vi "Set_PackedLibrary_Data.vi"(8 "error in (no error)":errorcluster, 10 "data":T1, 11 "Class in":refnum<class "AB_PackedLibrary.lvclass">) -> (0 "error out":errorcluster, 3 "Class out":refnum<class "AB_PackedLibrary.lvclass">)   [LabVIEW 2020, in "AB_PackedLibrary.lvclass"]
uses:
  <vilib>/AppBuilder/AB_Classes/PackedLib/AB_PackedLibrary.lvclass
  <vilib>/AppBuilder/AB_Classes/PackedLib/AB_PackedLibrary.ctl
  <vilib>/AppBuilder/AB_Classes/PackedLib/AB_PackedLibrary.lvclass/AB_PackedLibrary.ctl
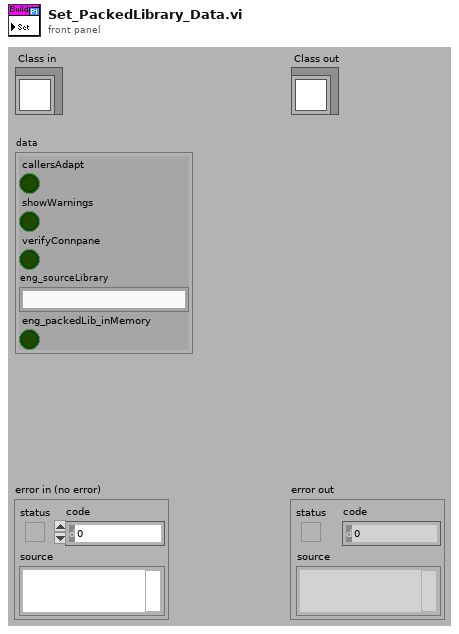
[diagram p1: front panel]
types:
  T1 = typedef "AB_PackedLibrary.ctl" = cluster{"callersAdapt":bool, "showWarnings":bool, "verifyConnpane":bool, "eng_sourceLibrary":string, "eng_packedLib_inMemory":bool}
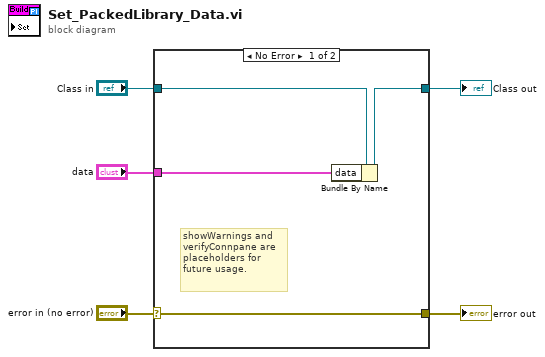
[diagram p0: block diagram]
diagram:
  n1 = case shown="No Error" "error in (no error)" {
    selector: "error in (no error)" -> [w9 w11]
    tunnel: [w9 w11] -> w4
    tunnel: [w6 w10] -> w3
    tunnel: "Class in" -> [w7 w10]
    tunnel: "data" -> [w8 _]
    frame No Error {
      # "showWarnings and verifyConnpane are placeholders for future usage."
      n2 = Bundle By Name(cluster=w7, "data"=w8) -> (w6:refnum<class "AB_PackedLibrary.lvclass">)
    }
    frame Error {
    }
  }
  "Class out" <- w3
  "error out" <- w4
